vi "LJM_MACToNumber.vi"(8 "error in":errorcluster, 10 "MACString":string="01:23:45:67:89:AB") -> (0 "error out":errorcluster, 1 "Number as 2 Integers":cluster{"Number MS32":u32, "Number LS32":u32}, 2 "Number Ext":ext format="%#.0f")   [LabVIEW 2020]
uses:
  LabJackM.framework
panel:
  # "A MAC of 01:23:45:67:89:AB equates to a number\nof 1250999896491.  Written as 2 U32 that is\nan MS32 of 291 and an LS32 of 1164413355."
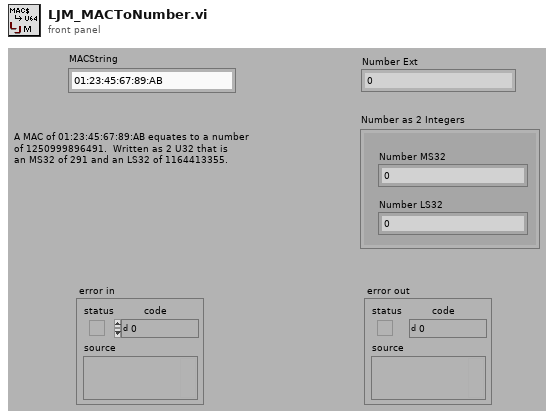
[diagram p1: front panel]
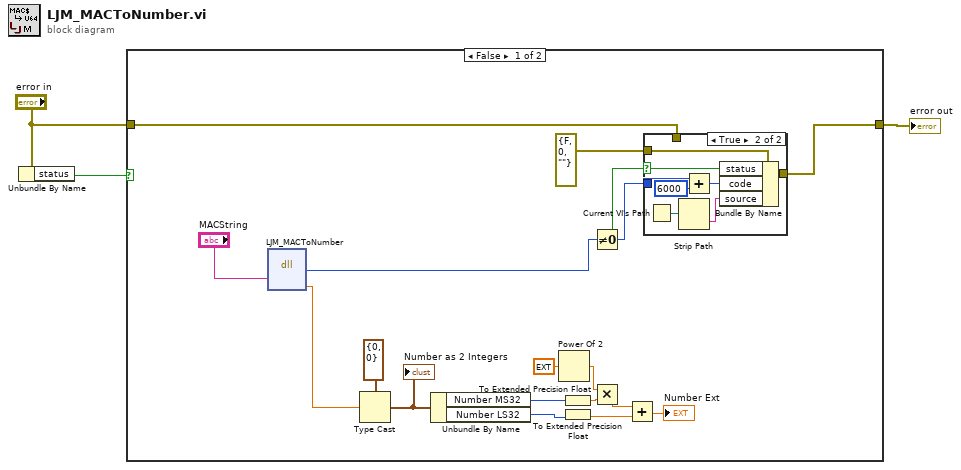
[diagram p0: block diagram]
diagram:
  n1 = Unbundle By Name("error in") -> ("status"=w3:bool)
  n2 = case shown="False" w3 {
    tunnel: "error in" -> [w17 w30]
    tunnel: [w16 w30] -> w1
    frame False {
      n3 = dll-call lib="LabJackM.framework" fn="LJM_MACToNumber"("MACString"="MACString") -> ("return type"=w20:i32, "Number"=w14:dbl)  [unwired: 5 in, 2 out]
      n4 = Type Cast(type=cluster{"Number MS32":u32, "Number LS32":u32} {"Number MS32"=0, "Number LS32"=0} ("Number as 2 Integers"), x=w14) -> (*(type *) &x=w5:cluster{"Number MS32":u32, "Number LS32":u32})
      "Number as 2 Integers" <- w5
      n5 = Unbundle By Name(w5) -> ("Number MS32"=w7:u32, "Number LS32"=w6:u32)
      n6 = Power Of 2(x=ext 32.0) -> (2^x=w11:ext)
      n7 = To Extended Precision Float(1:w7) -> (0:w12:ext)
      n8 = To Extended Precision Float(1:w6) -> (0:w8:ext)
      n9 = Not Equal To 0?(x=w20) -> (x != 0?=w19:bool)
      n10 = Multiply(x=w11, y=w12) -> (x*y=w10:ext)
      n11 = Add(x=w10, y=w8) -> (x+y=→"Number Ext":ext)
      n12 = case shown="True" w19 {
        selector: w19 -> [_ w28]
        tunnel: [w21 w29] -> w16
        tunnel: errorcluster {"status"=FALSE, "code"=0, "source"=""} ("error IO") -> [_ w27]
        tunnel: w20 -> [_ w23]
        tunnel: w17 -> [w21 _]
        frame False {
        }
        frame True {
          n13 = Current VI's Path() -> (path=w25:path)
          n14 = Strip Path(path=w25) -> (name=w26:string)  [unwired: 1 out]
          n15 = Add(x=w23, y=6000) -> (x+y=w24:i32)
          n16 = Bundle By Name(cluster=w27, "status"=w28, "code"=w24, "source"=w26) -> (w29:errorcluster)
        }
      }
    }
    frame True {
    }
  }
  "error out" <- w1
